vi "write_DACs.vi"(7 "converter box version":i16=1 min=1 max=2, 11 "DAC values in":T1={"DAC channel enable"={"ch0"=TRUE, "ch1"=TRUE, "ch2"=TRUE, "ch3"=TRUE, "ch4"=TRUE, "ch5"=TRUE, "ch6"=TRUE}, "DAC voltage"={"ch0"=0, "ch1"=0, "ch2"=0, "ch3"=0, "ch4"=0, "ch5"=0, "ch6"=0}, "offset"=0, "channel index"=0, "bit index"=0, "synch?"=FALSE, "DAC clock"=FALSE, "finished?"=FALSE} {"bit index" min=-1 max=17 step=1; "channel index" max=7 step=1; "offset" max=4095; "DAC voltage"."ch6" max=4095 step=1; "DAC voltage"."ch5" max=4095 step=1; "DAC voltage"."ch4" max=4095 step=1; "DAC voltage"."ch3" max=4095 step=1; "DAC voltage"."ch2" max=4095 step=1; "DAC voltage"."ch1" max=4095 step=1; "DAC voltage"."ch0" max=4095 step=1}) -> (3 "DAQ values out":T1={"DAC channel enable"={"ch0"=TRUE, "ch1"=TRUE, "ch2"=TRUE, "ch3"=TRUE, "ch4"=TRUE, "ch5"=TRUE, "ch6"=TRUE}, "DAC voltage"={"ch0"=0, "ch1"=0, "ch2"=0, "ch3"=0, "ch4"=0, "ch5"=0, "ch6"=0}, "offset"=0, "channel index"=0, "bit index"=0, "synch?"=FALSE, "DAC clock"=FALSE, "finished?"=FALSE} {"bit index" min=-1 max=17 step=1; "channel index" max=7 step=1; "offset" max=4095; "DAC voltage"."ch6" max=4095 step=1; "DAC voltage"."ch5" max=4095 step=1; "DAC voltage"."ch4" max=4095 step=1; "DAC voltage"."ch3" max=4095 step=1; "DAC voltage"."ch2" max=4095 step=1; "DAC voltage"."ch1" max=4095 step=1; "DAC voltage"."ch0" max=4095 step=1})   [LabVIEW 2010]
uses:
  common_typedefs/DAC_values_cluster.ctl
  common_typedefs/DAC_channel_enable_cluster.ctl
  common_typedefs/DAC_voltage_cluster.ctl
  <vilib>/eio/EIONode/EIONode.xnode
  <vilib>/rvi/eio/nirviEIOImplementation/nirviEIOImplementation.xnode
  <vilib>/rvi/eio/common/nirviEmuClasses.ctl
  <vilib>/rvi/eio/common/nirviEmuTemplateMethod_noerrors.vi
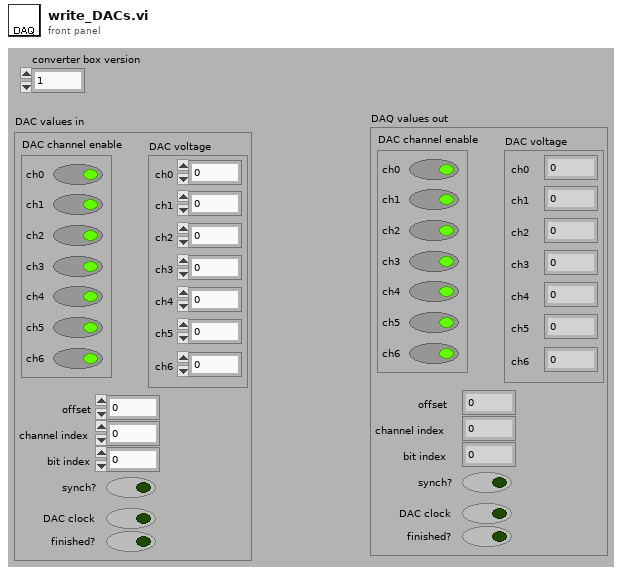
[diagram p1: front panel]
types:
  T1 = typedef "DAC_values_cluster.ctl" = cluster{"DAC channel enable":T2, "DAC voltage":T3, "offset":u16, "channel index":u16, "bit index":i32, "synch?":bool, "DAC clock":bool, "finished?":bool}
  T2 = typedef "DAC_channel_enable_cluster.ctl" = cluster{"ch0":bool, "ch1":bool, "ch2":bool, "ch3":bool, "ch4":bool, "ch5":bool, "ch6":bool}
  T3 = typedef "DAC_voltage_cluster.ctl" = cluster{"ch0":u16, "ch1":u16, "ch2":u16, "ch3":u16, "ch4":u16, "ch5":u16, "ch6":u16}
  T4 = typedef "nirviEmuClasses.ctl" = enum16{"IO Read", "IO Write", "Method", "Property Read", "Property Write"}
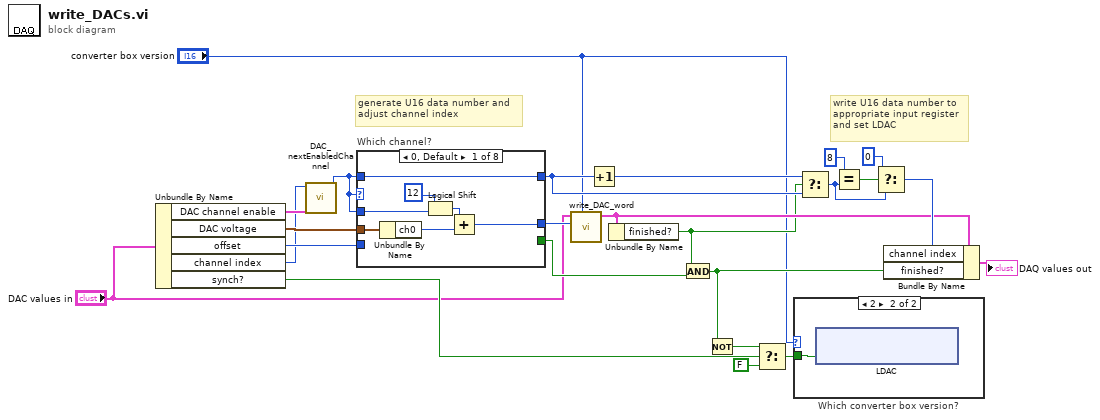
[diagram p0: block diagram]
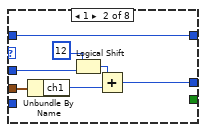
[diagram p3: hidden frame]
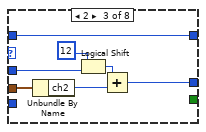
[diagram p4: hidden frame]
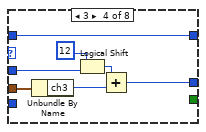
[diagram p5: hidden frame]
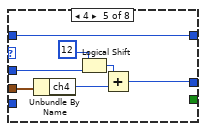
[diagram p6: hidden frame]
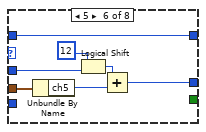
[diagram p7: hidden frame]
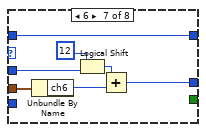
[diagram p8: hidden frame]
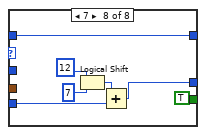
[diagram p9: hidden frame]
diagram:
  # "write U16 data number to\nappropriate input register\nand set LDAC"
  # "generate U16 data number and\nadjust channel index"
  n1 = Unbundle By Name("DAC values in") -> ("DAC channel enable"=w12:T2, "DAC voltage"=w11:T3, "offset"=w10:u16, "channel index"=w9:u16, "synch?"=w8:bool)
  n2 = call "DAC_nextEnabledChannel.vi"("DAC channel enable"=w12, "channel index in"=w9) -> ("nextEnabledChannelIndex"=w13:u16)  [unwired: 9 in]
  n3 = case "Which channel?" shown="0, Default" w13 {
    tunnel: w11 -> [w27 w38 w41 w48 w55 w62 w69 _]
    tunnel: w10 -> [_ _ _ _ _ _ _ w78]
    tunnel: w13 -> [w28 w35 w42 w49 w56 w63 w70 _]
    tunnel: [w25 w32 w39 w46 w53 w60 w67 w76] -> w24
    tunnel: [_ _ _ _ _ _ _ TRUE] -> w21
    tunnel: w13 -> [w26 w33 w40 w47 w54 w61 w68 w74]
    tunnel: [w26 w33 w40 w47 w54 w61 w68 w74] -> w19
    frame 0, Default {
      n4 = Unbundle By Name(w27) -> ("ch0"=w31:u16)
      n5 = Logical Shift(y=u16 12, x=w28) -> (x << y=w29:u16)
      n6 = Add(x=w29, y=w31) -> (x+y=w25:u16)
    }
    frame 1 {
      n7 = Unbundle By Name(w38) -> ("ch1"=w34:u16)
      n8 = Logical Shift(y=u16 12, x=w35) -> (x << y=w37:u16)
      n9 = Add(x=w37, y=w34) -> (x+y=w32:u16)
    }
    frame 2 {
      n10 = Unbundle By Name(w41) -> ("ch2"=w45:u16)
      n11 = Logical Shift(y=u16 12, x=w42) -> (x << y=w43:u16)
      n12 = Add(x=w43, y=w45) -> (x+y=w39:u16)
    }
    frame 3 {
      n13 = Unbundle By Name(w48) -> ("ch3"=w52:u16)
      n14 = Logical Shift(y=u16 12, x=w49) -> (x << y=w50:u16)
      n15 = Add(x=w50, y=w52) -> (x+y=w46:u16)
    }
    frame 4 {
      n16 = Unbundle By Name(w55) -> ("ch4"=w59:u16)
      n17 = Logical Shift(y=u16 12, x=w56) -> (x << y=w57:u16)
      n18 = Add(x=w57, y=w59) -> (x+y=w53:u16)
    }
    frame 5 {
      n19 = Unbundle By Name(w62) -> ("ch5"=w66:u16)
      n20 = Logical Shift(y=u16 12, x=w63) -> (x << y=w64:u16)
      n21 = Add(x=w64, y=w66) -> (x+y=w60:u16)
    }
    frame 6 {
      n22 = Unbundle By Name(w69) -> ("ch6"=w73:u16)
      n23 = Logical Shift(y=u16 12, x=w70) -> (x << y=w71:u16)
      n24 = Add(x=w71, y=w73) -> (x+y=w67:u16)
    }
    frame 7 {
      n25 = Logical Shift(y=u16 12, x=u16 7) -> (x << y=w79:u16)
      n26 = Add(x=w79, y=w78) -> (x+y=w76:u16)
    }
  }
  n27 = call "write_DAC_word.vi"("converter box version"="converter box version", "U16 data number"=w24, "DAC values in"="DAC values in") -> ("DAC values out"=w3:T1)  [unwired: 8 in]
  n28 = Increment(x=w19) -> (x+1=w18:u16)
  n29 = Unbundle By Name(w3) -> ("finished?"=w2:bool)
  n30 = And(x=w2, y=w21) -> (x .and. y?=w7:bool)
  n31 = Not(x=w7) -> (.not. x?=w20:bool)
  n32 = Select(t=w20, s=w8, f=FALSE) -> (s? t:f=w22:bool)
  n33 = case "Which converter box version?" shown="2" "converter box version" {
    tunnel: w22 -> [_ w81]
    frame Default {
    }
    frame 2 {
      n34 = xnode "LDAC"("Connector1/DIO32"=w81) -> ()  [unwired: 1 in, 1 out]
    }
  }
  n35 = Select(t=w18, s=w2, f=w19) -> (s? t:f=w14:u16)
  n36 = Equal?(x=u16 8, y=w14) -> (x = y?=w16:bool)
  n37 = Select(t=u16 0, s=w16, f=w14) -> (s? t:f=w6:u16)
  n38 = Bundle By Name(cluster=w3, "channel index"=w6, "finished?"=w7) -> (→"DAQ values out":T1)
